vi "GetPredecessors.vi"(8 "error in (no error)":errorcluster, 10 "NodeReference":refnum<data-value>, 11 "WorldMap in":refnum<class "NI_Robotics_DirectedGraphWorldMap.lvclass">) -> (0 "error out":errorcluster, 1 "EdgeCost":dbl[](array[numeric]), 2 "Predecessors":refnum<data-value>[](array[refnum]), 3 "WorldMap out":refnum<class "NI_Robotics_DirectedGraphWorldMap.lvclass">)   [LabVIEW 2017, in "NI_Robotics_DirectedGraphWorldMap.lvclass"]
uses:
  <vilib>/robotics/Navigation/shared/WorldMap/DirectedGraphWorldMap/NI_Robotics_DirectedGraphWorldMap.lvclass
  <vilib>/robotics/Navigation/shared/MapNode/AbstractMapNode/NI_Robotics_AbstractMapNode.lvclass
  <vilib>/robotics/Navigation/shared/MapNode/DirectedGraphMapNode/NI_Robotics_DirectedGraphMapNode.lvclass
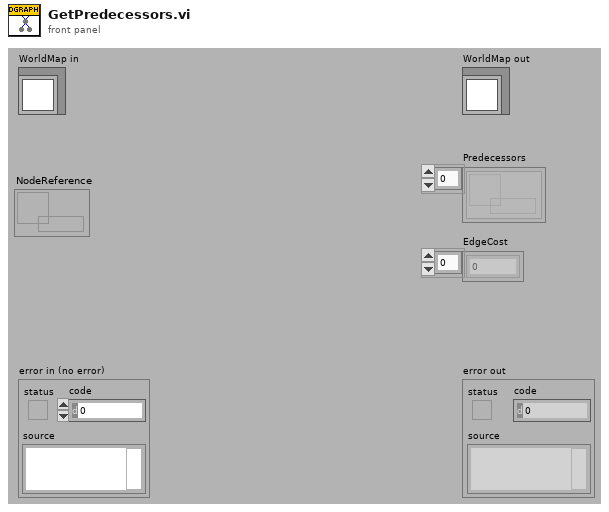
[diagram p1: front panel]
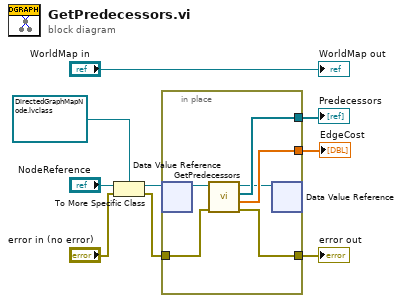
[diagram p0: block diagram]
diagram:
  n1 = To More Specific Class(target class=refnum<data-value> refnum ("data value reference"), reference="NodeReference", error in="error in (no error)") -> (specific class reference=w4:refnum<data-value>, error out=w1:errorcluster)
  n2 = in-place {
    in-place-border: w1 -> [w10]
    in-place-border: [w15] -> w8
    in-place-border: [w14] -> w7
    in-place-border: [w13] -> w6
    n3 = in-place-dvr #1(w4) -> (w12:refnum<class "NI_Robotics_DirectedGraphMapNode.lvclass">)  [unwired: 1 out]
    n4 = call-dynamic "GetPredecessors.vi"("error in (no error)"=w10, "DirectedGraphMapNode in"=w12) -> ("error out"=w15:errorcluster, "Predecessor Costs"=w13:dbl[], "Predecessors"=w14:refnum<data-value>[], "DirectedGraphMapNode out"=w11:refnum<class "NI_Robotics_DirectedGraphMapNode.lvclass">)  [unwired: 6 in]
    n5 = in-place-dvr #1(w11) -> ()  [unwired: 2 out]
  }
  "error out" <- w8
  "EdgeCost" <- w6
  "Predecessors" <- w7
  "WorldMap out" <- "WorldMap in"
